vi "Delete row item.vi"(11 "Data Cluster in":T1 {"Pump_data"."mix rpm" format="%.2f"; "Pump_data"."Volume corrected" format="%.2f"; "Pump_data"."Position_MM" format="%.3f"; "Pump_data"."Volume PV" format="%.2f"; "Pump_data"."Flow PV" format="%#.6f"; "Pump_data"."Pressure PV" format="%.3f"}) -> (0 "error out":errorcluster, 1 "Ok?":bool, 2 "New P":dbl, 3 "Data Cluster out":T1 {"Pump_data"."mix rpm" format="%.2f"; "Pump_data"."Volume corrected" format="%.2f"; "Pump_data"."Position_MM" format="%.3f"; "Pump_data"."Volume PV" format="%.2f"; "Pump_data"."Flow PV" format="%#.6f"; "Pump_data"."Pressure PV" format="%.3f"})   [LabVIEW 2023, in "AutoPV.lvlib"]
uses:
  AutoPV.lvlib
  Module Data--cluster.ctl
  <vilib>/ActorFramework/Message Enqueuer/Message Enqueuer.lvclass
  Drive/Pump_Data_Type.ctl
  Initial Data/InitalData Type.ctl
  Drive/Drive.lvlib
  Initial Data/Initial Data.lvlib
panel:
  # "Образец"
  # "Образец"
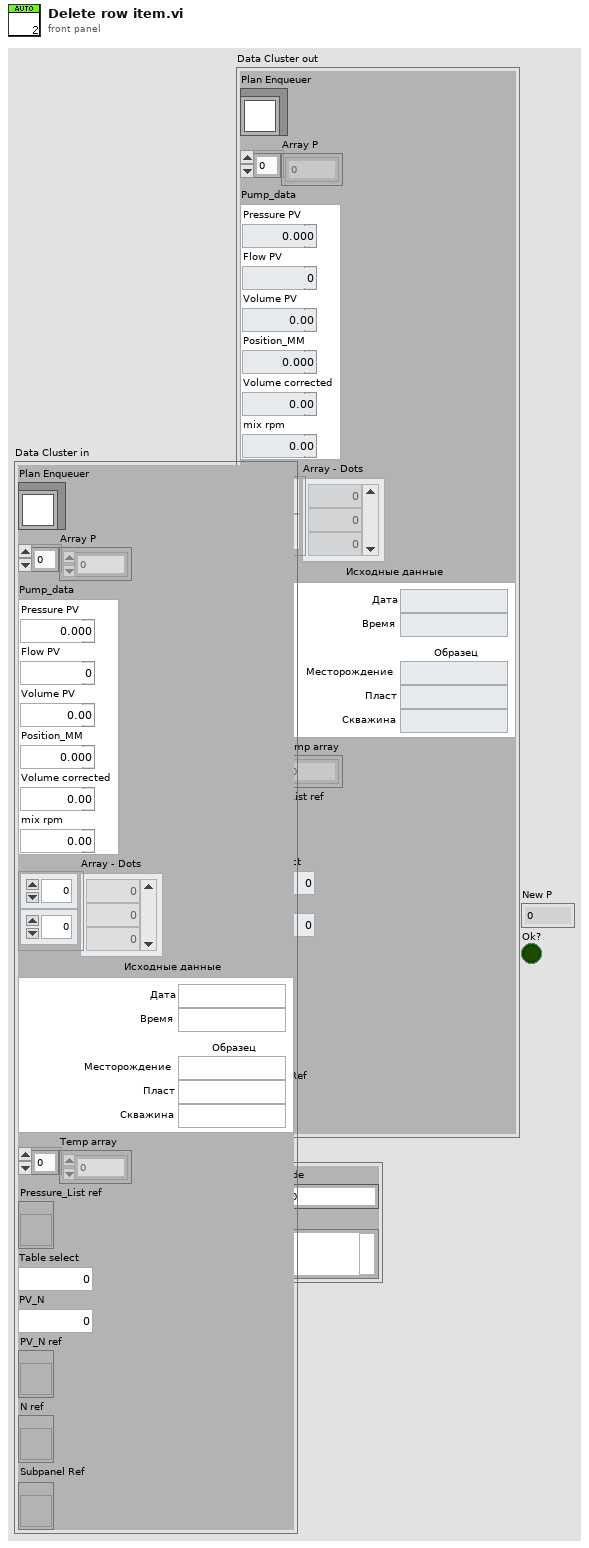
[diagram p1: front panel]
types:
  T1 = typedef "AutoPV.lvlib/Module Data--cluster.ctl" = cluster{"Plan Enqueuer":refnum<class "Message Enqueuer.lvclass">, "Array P":dbl[], "Pump_data":T2, "Array - Dots":dbl[][], "Исходные данные":T3, "Temp array":dbl[], "Pressure_List ref":refnum<vi>, "Table select":i32, "PV_N":i32, "PV_N ref":refnum<vi>, "N ref":refnum<vi>, "Subpanel Ref":refnum<vi>}
  T2 = typedef "Drive.lvlib/Pump_Data_Type.ctl" = cluster{"Pressure PV":dbl, "Flow PV":dbl, "Volume PV":dbl, "Position_MM":dbl, "Volume corrected":dbl, "mix rpm":dbl}
  T3 = typedef "Initial Data.lvlib/InitalData Type.ctl" = cluster{"Дата":string, "Время":string, "Месторождение":string, "Пласт":string, "Скважина":string}
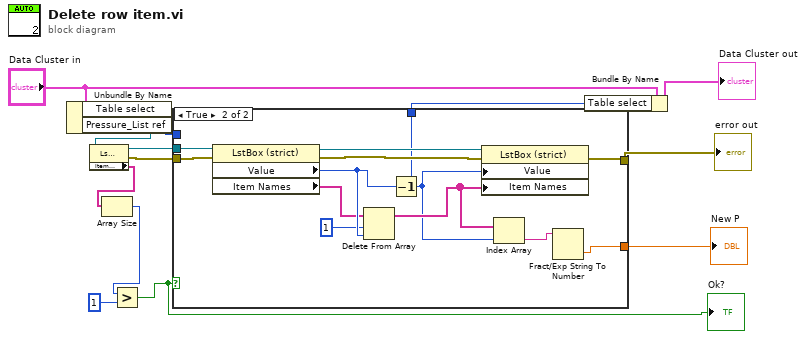
[diagram p0: block diagram]
diagram:
  n1 = Unbundle By Name("Data Cluster in") -> ("Table select"=w13:i32, "Pressure_List ref"=w5:refnum<vi>)
  n2 = property class="LstBox (strict)"(reference=w5) -> (reference out=w6:refnum<vi>, error out=w7:errorcluster, "Item Names"=w8:string[])  [unwired: 1 in]
  n3 = Array Size(array=w8) -> (size(s)=w9:i32)
  n4 = Greater?(x=w9, y=1) -> (0:w1:bool)
  "Ok?" <- w1
  n5 = case shown="True" w1 {
    tunnel: w6 -> [_ w27]
    tunnel: [w15 w26] -> w4
    tunnel: w7 -> [w15 w21]
    tunnel: [w14 w18] -> w12
    tunnel: w13 -> [w14 _]
    tunnel: [_ w16] -> w2
    frame False {
    }
    frame True {
      n6 = property class="LstBox (strict)"(reference=w27, error in=w21) -> (reference out=w25:refnum<vi>, error out=w20:errorcluster, "Value"=w24:i32, "Item Names"=w23:string[])
      n7 = Delete From Array(array=w23, length=1, index=w24) -> (array with subset deleted=w19:string[])  [unwired: 1 out]
      n8 = Decrement(x=w24) -> (x-1=w18:i32)
      n9 = property class="LstBox (strict)"(reference=w25, error in=w20, "Value"=w18, "Item Names"=w19) -> (error out=w26:errorcluster)  [unwired: 1 out]
      n10 = Index Array(array=w19, index=w18) -> (element=w17:string)
      n11 = Fract/Exp String To Number(string=w17) -> (number=w16:dbl)  [unwired: 3 in, 1 out]
    }
  }
  "error out" <- w4
  "New P" <- w2
  n12 = Bundle By Name(cluster="Data Cluster in", "Table select"=w12) -> (→"Data Cluster out":T1)
